vi "PCA9586-Servo_Test.vi"() -> ()   [LabVIEW 2019]
panel:
  out "當前角度":dbl
  in  "角度":dbl(slide) scale=0.0..180.0
  in  "Stop":bool
  in  "PWM腳位":T1(ring)
  in  "Error In":errorcluster
  out "Error Out":errorcluster
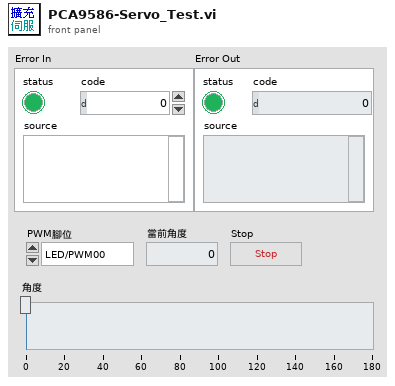
[diagram p1: front panel]
types:
  T1 = enum16{"LED/PWM00", "LED/PWM01", "LED/PWM02", "LED/PWM03", "LED/PWM04", "LED/PWM05", "LED/PWM06", "LED/PWM07", "LED/PWM08", "LED/PWM09", "LED/PWM10", "LED/PWM11", "LED/PWM12", "LED/PWM13", "LED/PWM14", "LED/PWM15"}
  T2 = typedef "I2C.lvlib/I2C Reference.ctl" = cluster{"myRIO Reference":T3, "I2C Channels Enum":T7, "I2C Configuration":T8}
  T3 = typedef "myRIO Generic Hardware Reference.ctl" = cluster{"myRIO Model":T4, "myRIO Hardware Reference":T5}
  T4 = typedef "Hardware Version Enum.ctl" = enum16{"Unknown", "myRIO-1900", "myRIO-1950", "roboRIO", "NI ELVIS RIO CM", "ELVIS III"}
  T5 = typedef "myRIO v1.0 Reference.ctl" = cluster{"Generic FPGA Reference":T6, "Allow multiple opens":bool}
  T6 = typedef "Generic FPGA Reference.ctl" = refnum<k20>
  T7 = typedef "I2C Channels Enum.ctl" = enum16{"Not Connected", "A/I2C", "B/I2C", "I2C/I2C"}
  T8 = typedef "I2C.lvlib/I2C Configuration.ctl" = cluster{"I2C Transfer Rate":T9}
  T9 = typedef "I2C.lvlib/I2C Transfer Rate.ctl" = enum16{"Standard mode (100 kbps)", "Fast mode (400 kbps)"}
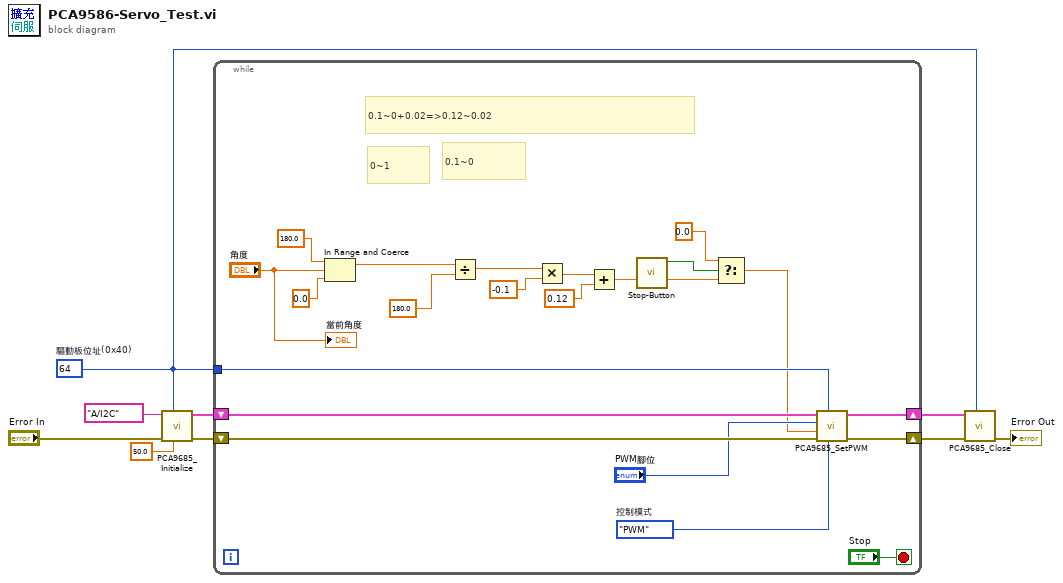
[diagram p0: block diagram]
diagram:
  w1 = u8 64  # 驅動板位址(0x40)
  n1 = call "PCA9685_Initialize.vi"("PWM頻率(50Hz)"=50.0, "驅動板位址(0x40)"=w1, "Error In"="Error In", "I2C腳位"=tag "A/I2C") -> ("Error Out"=w5:errorcluster, "I2C Ref Out"=w9:T2)  [unwired: 6 in]
  n2 = while {
    tunnel: w1 -> [w24]
    shift-right: [w29] -> w8
    shift-left: w9 -> [w30]
    shift-right: [w28] -> w7
    shift-left: w5 -> [w27]
    stop <- "Stop" stop-if-true
    w26 = enum16{"PWM", "LED ON", "LED OFF"}."PWM"  # 控制模式
    # "0.1~0+0.02=>0.12~0.02"
    # "0.1~0"
    # "0~1"
    n3 = In Range and Coerce(upper limit=180.0, x="角度", lower limit=0.0) -> (coerced(x)=w21:dbl)  [unwired: 1 out]
    n4 = Divide(x=w21, y=180.0) -> (x/y=w19:dbl)
    n5 = Multiply(x=w19, y=-0.1) -> (x*y=w17:dbl)
    n6 = Add(x=w17, y=0.12) -> (x+y=w15:dbl)
    n7 = call "Stop-Button.vi"() -> ("顯示按下?"=w13:bool)  [unwired: 10 in, 1 out]
    n8 = Select(t=0.0, s=w13, f=w15) -> (s? t:f=w12:dbl)
    n9 = call "PCA9685_SetPWM.vi"("控制模式"=w26, "驅動板位址(0x40)"=w24, "Error In"=w27, "Duty Cycle(0~1)"=w12, "PWM腳位"="PWM腳位", "I2C Ref In"=w30) -> ("Error Out"=w28:errorcluster, "I2C Ref Out"=w29:T2)  [unwired: 4 in]
    "當前角度" <- "角度"
  }
  n10 = call "PCA9685_Close.vi"("驅動板位址(0x40)"=w1, "Error In"=w7, "I2C Ref In"=w8) -> ("Error Out"=→"Error Out":errorcluster)  [unwired: 8 in]
